vi "Init.vi"(8 "error in (no error)":errorcluster, 10 "Value":i64=-1, 11 "Depth":i32) -> (0 "error out":errorcluster, 3 "SnailNum out":refnum<class "SnailNum.lvclass">)   [LabVIEW 2020, in "SnailNum.lvclass"]
uses:
  SnailNum.lvclass
  SnailNum.lvclass/SnailNum.ctl
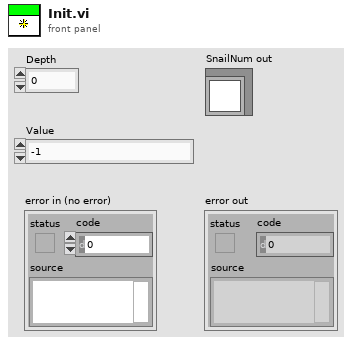
[diagram p1: front panel]
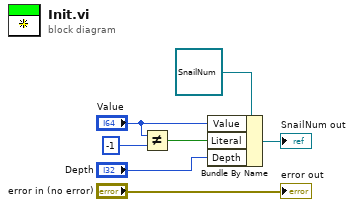
[diagram p0: block diagram]
diagram:
  n1 = Not Equal?(x="Value", y=i64 -1) -> (x != y?=w2:bool)
  n2 = Bundle By Name(cluster=refnum<class "SnailNum.lvclass"> refnum ("SnailNum in"), "Value"="Value", "Literal"=w2, "Depth"="Depth") -> (→"SnailNum out":refnum<class "SnailNum.lvclass">)
  "error out" <- "error in (no error)"
